vi "XY_scanner3.vi"(3 "offset Y":dbl, 5 "offset X":dbl, 6 "Line_start":i32, 7 "Range":dbl=10.0, 8 "Pixels":i32=256, 9 "dwell":dbl=1.0) -> (0 "X and Y":waveform(dbl)[](array[waveform]), 1 "Array Y":dbl[](array[numeric]), 2 "Array X":dbl[](array[numeric]), 4 "scanPix":i32)   [LabVIEW 2016]
panel:
  out "Waveform Graph 3":waveform(dbl)[](graph)
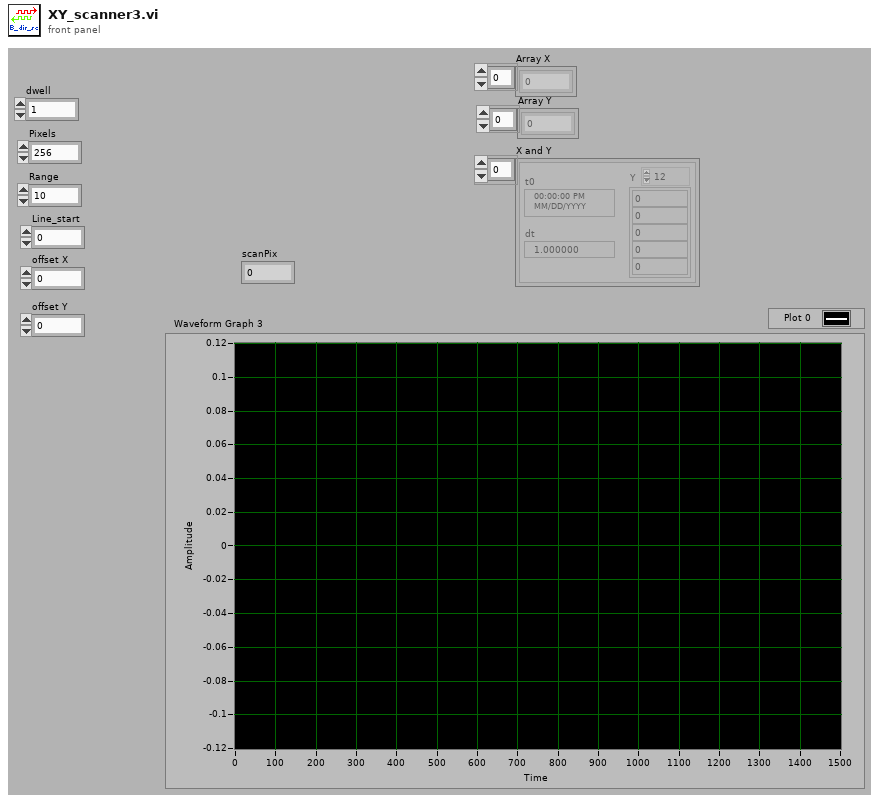
[diagram p1: front panel]
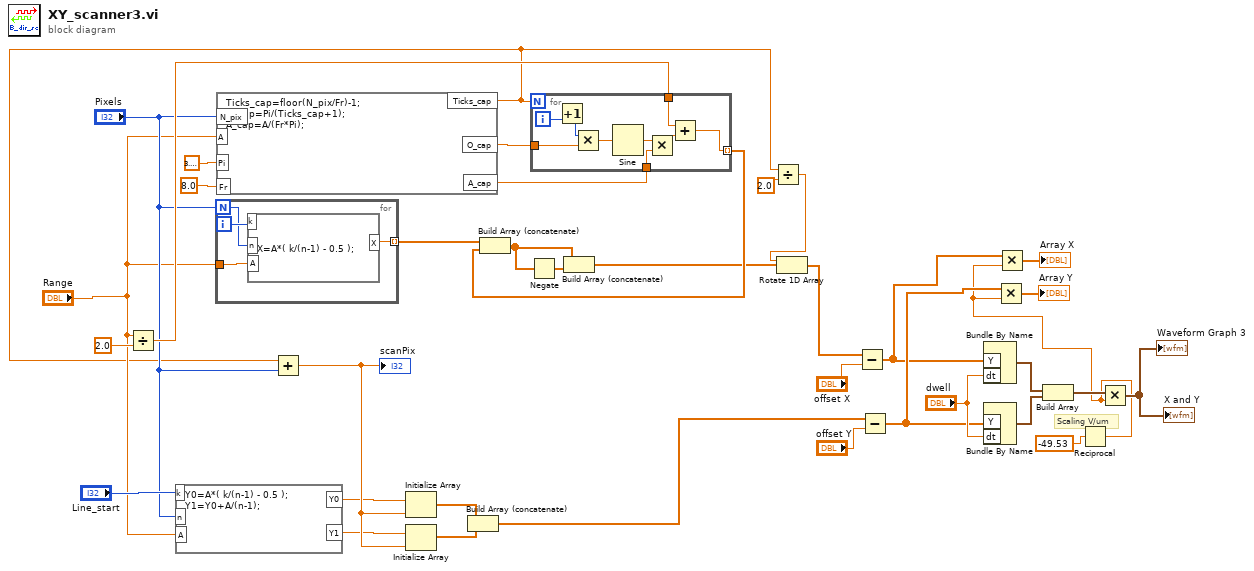
[diagram p0: block diagram]
diagram:
  # "Scaling V/um"
  n1 = Divide(x="Range", y=2.0) -> (x/y=w21:dbl)
  n2 = formula code="Y0=A*( k/(n-1) - 0.5 );\nY1=Y0+A/(n-1);"("k"="Line_start", "n"="Pixels", "A"="Range") -> ("Y0"=w15:dbl, "Y1"=w14:dbl)
  n3 = for {
    N: "Pixels" -> [w39]
    tunnel: [w41] -> w22 mode=indexing
    tunnel: "Range" -> [w38]
    i -> [w40]
    n4 = formula code="X=A*( k/(n-1) - 0.5 );"("k"=w40, "n"=w39, "A"=w38) -> ("X"=w41:dbl)
  }
  n5 = formula code="Ticks_cap=floor(N_pix/Fr)-1;\nO_cap=Pi/(Ticks_cap+1);\nA_cap=A/(Fr*Pi);"("N_pix"="Pixels", "A"="Range", "Fr"=8.0 ("input variable"), "Pi"=3.141592653589793) -> ("Ticks_cap"=w1:dbl, "A_cap"=w27:dbl, "O_cap"=w25:dbl)
  n6 = Add(x=w1, y="Pixels") -> (x+y=w35:dbl)
  "scanPix" <- w35
  n7 = Initialize Array(w15, w35) -> (w13:dbl[])
  n8 = Initialize Array(w14, w35) -> (w34:dbl[])
  n9 = Build Array (concatenate)(w13, w34) -> (w24:dbl[])
  n10 = for {
    N: w1 -> [_]
    tunnel: [w44] -> w26 mode=indexing
    tunnel: w27 -> [w47]
    tunnel: w25 -> [w42]
    tunnel: w21 -> [w45]
    i -> [w50]
    n11 = Increment(x=w50) -> (x+1=w43:i32)
    n12 = Multiply(x=w43, y=w42) -> (x*y=w49:dbl)
    n13 = Sine(x=w49) -> (sin(x)=w48:dbl)
    n14 = Multiply(x=w48, y=w47) -> (x*y=w46:dbl)
    n15 = Add(x=w45, y=w46) -> (x+y=w44:dbl)
  }
  n16 = Build Array (concatenate)(w22, w26) -> (w19:dbl[])
  n17 = Negate(x=w19) -> (-x=w20:dbl[])
  n18 = Build Array (concatenate)(w19, w20) -> (w12:dbl[])
  n19 = Divide(x=w1, y=2.0) -> (x/y=w10:dbl)
  n20 = Rotate 1D Array(1:w12, 2:w10) -> (0:w11:dbl[])
  n21 = Subtract(x=w11, y="offset X") -> (x-y=w5:dbl[])
  n22 = Subtract(x=w24, y="offset Y") -> (x-y=w6:dbl[])
  n23 = Bundle By Name("Y"=w5, "dt"="dwell") -> (w31:waveform(dbl))  [unwired: 1 in]
  n24 = Bundle By Name("Y"=w6, "dt"="dwell") -> (w30:waveform(dbl))  [unwired: 1 in]
  n25 = Build Array(w31, w30) -> (w23:waveform(dbl)[])
  n26 = Reciprocal(x=-49.53 ("y")) -> (1/x=w4:dbl)
  n27 = Multiply(x=w6, y=w4) -> (x*y=→"Array Y":dbl[])
  n28 = Multiply(x=w5, y=w4) -> (x*y=→"Array X":dbl[])
  n29 = Multiply(x=w23, y=w4) -> (x*y=→"X and Y" →"Waveform Graph 3":waveform(dbl)[])
